vi "setFilterFrequencies.vi"(4 "mainLoopFrequency":sgl, 5 "cutoffMagneto":sgl, 6 "cutoffAccel":sgl, 7 "cutoffGyro":sgl, 8 "error in (no error)":errorcluster, 9 "gyroAccelsSampling":sgl, 11 "pHandle":u32) -> (0 "error out":errorcluster, 3 "return type":i32)   [LabVIEW 2011, in "sbgLabView.lvlib"]
uses:
  sbgLabView.lvlib
  sbgMatLab.dll
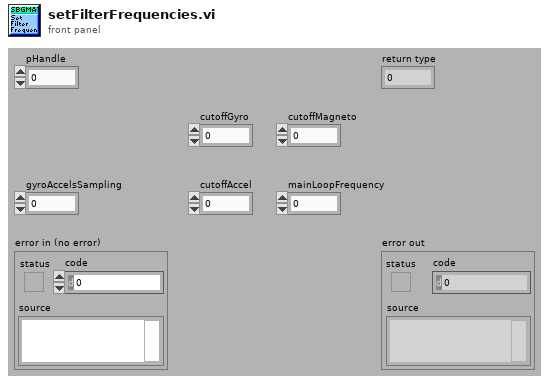
[diagram p1: front panel]
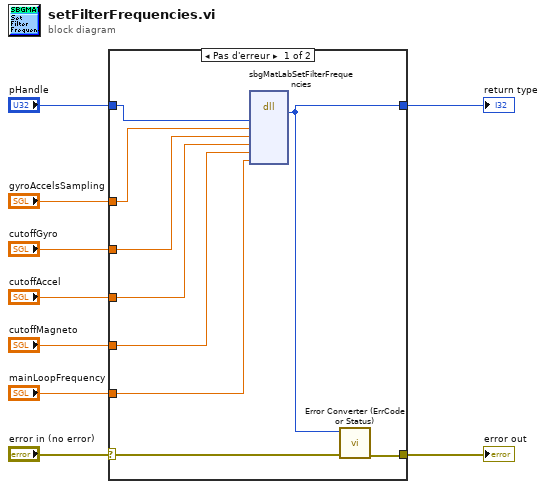
[diagram p0: block diagram]
diagram:
  n1 = case shown="Pas d'erreur" "error in (no error)" {
    selector: "error in (no error)" -> [w16 w19]
    tunnel: [w15 w19] -> w8
    tunnel: [w18 _] -> w7
    tunnel: "pHandle" -> [w17 _]
    tunnel: "gyroAccelsSampling" -> [w14 _]
    tunnel: "cutoffGyro" -> [w13 _]
    tunnel: "cutoffAccel" -> [w12 _]
    tunnel: "cutoffMagneto" -> [w11 _]
    tunnel: "mainLoopFrequency" -> [w10 _]
    frame No Error {
      n2 = dll-call lib="C:/SBG-Systems/remote/projects/software/projects/labviewExample/sbgLabView/sbgMatLab.*" fn="sbgMatLabSetFilterFrequencies"("pHandle"=w17, "gyroAccelsSampling"=w14, "cutoffGyro"=w13, "cutoffAccel"=w12, "cutoffMagneto"=w11, "mainLoopFrequency"=w10) -> ("return type"=w18:i32)  [unwired: 9 in, 2 out]
      n3 = call "Error Converter (ErrCode or Status).vi"("error in (no error)"=w16, "error code"=w18) -> ("error out"=w15:errorcluster)  [unwired: 9 in]
    }
    frame Error {
    }
  }
  "return type" <- w7
  "error out" <- w8
